vi "Configure Multi-Carrier Power Carriers.vi"(0 "VISA resource name":refnum<visa-resource-name>, 1 "Enable Auto Reference Carrier Frequency (T: Enable)":bool=TRUE, 2 "Manual Reference Carrier Frequency (1E+9Hz)":dbl=1000000000.0 format="%#.6g", 5 "Carriers Count (4)":i32=4, 7 "Enable Auto Reference Carrier (T: Enable)":bool=TRUE, 9 "Manual Reference Carrier (10)":i32=10, 11 "error in (no error)":errorcluster, 12 "Carrier Power Present":bool[](array[boolean])=[TRUE, TRUE], 13 "Carrier Width":dbl[](array[numeric])=[5000000.0, 5000000.0] format="%#.6g", 14 "Carrier Integration Bandwidth":dbl[](array[numeric])=[3800000.0, 3800000.0] format="%#.6g") -> (4 "VISA resource name out":refnum<visa-resource-name>, 15 "error out":errorcluster)   [LabVIEW 2014, in "Agilent ESA PSA Series.lvlib"]
doc: "Configures carriers. \n\n<B>Note:</B> \n\nThis VI is only usefuk when the measurement is set to Multi Carrier Power."
uses:
  Agilent ESA PSA Series.lvlib
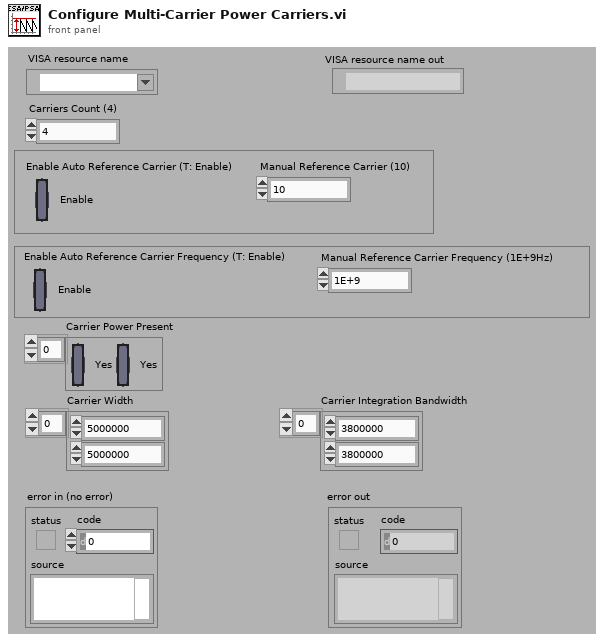
[diagram p1: front panel]
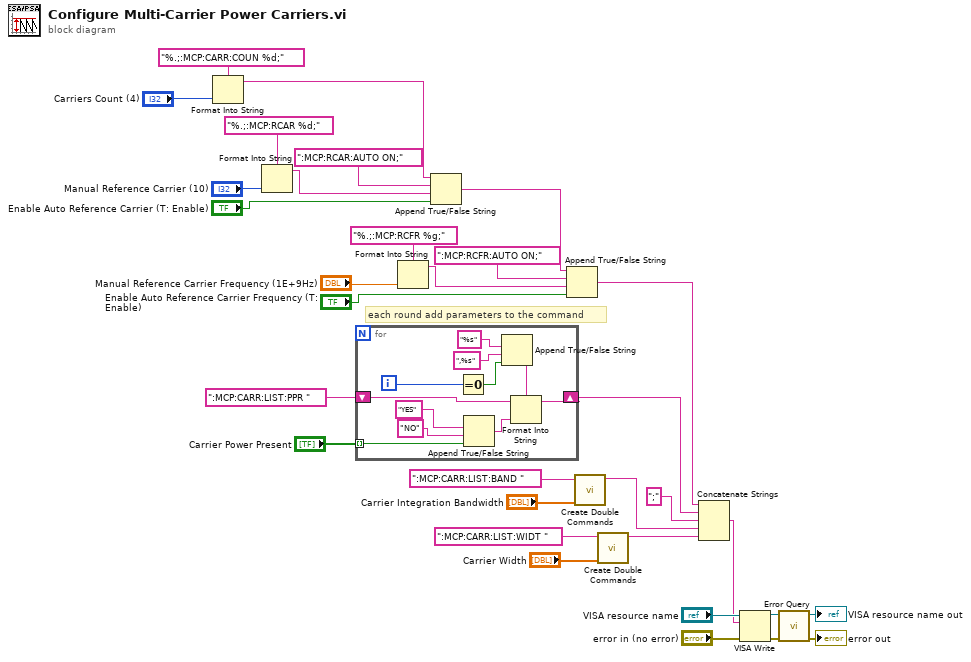
[diagram p0: block diagram]
diagram:
  # "each round add parameters to the command"
  n1 = Format Into String(format string="%.;:MCP:CARR:COUN %d;", "Carriers Count (4)") -> (resulting string=w8:string)  [unwired: 2 in, 1 out]
  n2 = Format Into String(format string="%.;:MCP:RCAR %d;", "Manual Reference Carrier (10)") -> (resulting string=w12:string)  [unwired: 2 in, 1 out]
  n3 = for {
    shift-right: [w34] -> w17
    shift-left: ":MCP:CARR:LIST:PPR " -> [w35]
    tunnel: "Carrier Power Present" -> [w33] mode=indexing
    i -> [w36]
    n4 = Equal To 0?(x=w36) -> (x = 0?=w37:bool)
    n5 = Append True/False String(1:w33, 2:"NO" ("false string"), 3:"YES" ("true string")) -> (0:w42:string)  [unwired: 1 in]
    n6 = Append True/False String(1:w37, 2:",%s" ("format string"), 3:"%s" ("format string")) -> (0:w43:string)  [unwired: 1 in]
    n7 = Format Into String(format string=w43, initial string=w35, w42) -> (resulting string=w34:string)  [unwired: 1 in, 1 out]
  }
  n8 = Format Into String(format string="%.;:MCP:RCFR %g;", "Manual Reference Carrier Frequency (1E+9Hz)") -> (resulting string=w6:string)  [unwired: 2 in, 1 out]
  n9 = Append True/False String(1:"Enable Auto Reference Carrier (T: Enable)", 2:w12, 3:":MCP:RCAR:AUTO ON;" ("initial string"), 4:w8) -> (0:w2:string)
  n10 = Append True/False String(1:"Enable Auto Reference Carrier Frequency (T: Enable)", 2:w6, 3:":MCP:RCFR:AUTO ON;" ("initial string"), 4:w2) -> (0:w1:string)
  n11 = call "Create Double Commands.vi"("Double Values"="Carrier Integration Bandwidth", "Commands"=":MCP:CARR:LIST:BAND ") -> ("Result"=w21:string)  [unwired: 9 in]
  n12 = call "Create Double Commands.vi"("Double Values"="Carrier Width", "Commands"=":MCP:CARR:LIST:WIDT ") -> ("Result"=w20:string)  [unwired: 9 in]
  n13 = Concatenate Strings(w1, w17, ";" ("string"), w21, w20) -> (w26:string)
  n14 = VISA Write(VISA resource name="VISA resource name", write buffer=w26, error in (no error)="error in (no error)") -> (VISA resource name out=w31:refnum<visa-resource-name>, error out=w32:errorcluster)  [unwired: 1 out]
  n15 = call "Error Query.vi"("error in (no error)"=w32, "VISA resource name"=w31) -> ("error out"=→"error out":errorcluster, "VISA resource name out"=→"VISA resource name out":refnum<visa-resource-name>)  [unwired: 6 in, 2 out]
